vi "Send_ZMQ_REQ_Multi.vi"(6 "timeout (ms)":u32=500, 7 "endpoint":string="tcp://127.0.0.1:5555", 8 "error in":errorcluster, 10 "Data in":string[](array[string])) -> (0 "error out":errorcluster, 1 "timeout?":bool, 2 "Reply":string[](array[string]))   [LabVIEW 2019, in "mmW_commands.lvlib"]
uses:
  mmW_commands.lvlib
  <vilib>/addons/zeromq/socket_type.ctl
  <vilib>/addons/zeromq/zeromq.lvlib
  <vilib>/addons/zeromq/zmq_context.lvclass
  <vilib>/addons/zeromq/zmq_socket.lvclass
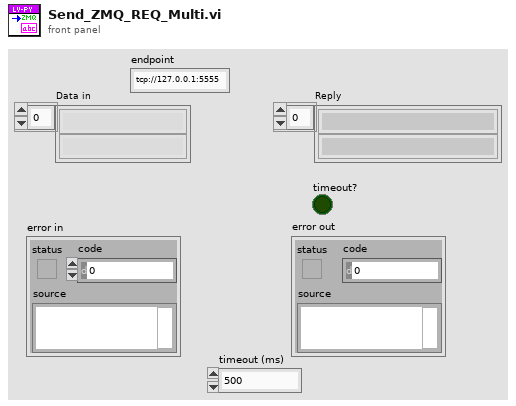
[diagram p1: front panel]
types:
  T1 = typedef "zeromq.lvlib/socket_type.ctl" = enum8{"ZMQ_PAIR", "ZMQ_PUB", "ZMQ_SUB", "ZMQ_REQ", "ZMQ_REP", "ZMQ_DEALER", "ZMQ_ROUTER", "ZMQ_PULL", "ZMQ_PUSH", "ZMQ_XPUB", "ZMQ_XSUB"}
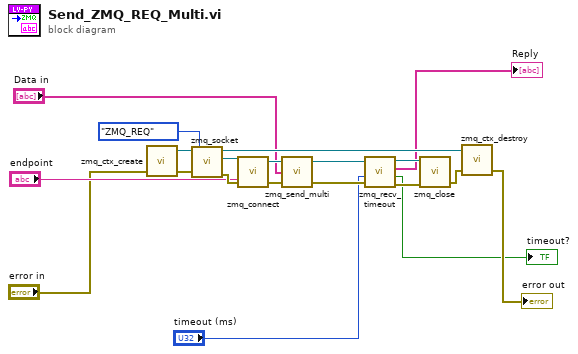
[diagram p0: block diagram]
diagram:
  n1 = call <vilib>:"zmq_ctx_create.vi"("error in"="error in") -> ("error out"=w10:errorcluster, "context out"=w20:refnum<class "zmq_context.lvclass">)  [unwired: 3 in]
  n2 = call <vilib>:"zmq_socket.vi"("error in"=w10, "socket type"=socket_type."ZMQ_REQ", "context in"=w20) -> ("error out"=w19:errorcluster, "socket out"=w18:refnum<class "zmq_socket.lvclass">, "context out"=w11:refnum<class "zmq_context.lvclass">)  [unwired: 2 in]
  n3 = call <vilib>:"zmq_connect.vi"("error in"=w19, "endpoint"="endpoint", "socket in"=w18) -> ("error out"=w17:errorcluster, "socket out"=w16:refnum<class "zmq_socket.lvclass">)  [unwired: 1 in]
  n4 = call <vilib>:"zmq_send_multi.vi"("error in"=w17, "parts"="Data in", "socket in"=w16) -> ("error out"=w9:errorcluster, "socket out"=w15:refnum<class "zmq_socket.lvclass">)  [unwired: 1 in]
  n5 = call <vilib>:"zmq_recv_timeout.vi"("error in"=w9, "timeout (ms)"="timeout (ms)", "socket in"=w15) -> ("error out"=w14:errorcluster, "timeout?"=→"timeout?":bool, "parts"=→"Reply":string[], "socket out"=w13:refnum<class "zmq_socket.lvclass">)  [unwired: 1 in]
  n6 = call <vilib>:"zmq_close.vi"("error in"=w14, "socket"=w13) -> ("error out"=w12:errorcluster)  [unwired: 3 in]
  n7 = call <vilib>:"zmq_ctx_destroy.vi"("error in"=w12, "context in"=w11) -> ("error out"=→"error out":errorcluster)  [unwired: 3 in]
